vi "Bit Array to Number.vi"(0 "Bit 0":bool, 5 "Bit 1":bool, 7 "Bit 2":bool) -> (8 "flags":u16)   [LabVIEW 2014]
panel:
  # "Copyright 2014 Vidrio Technologies\nScanImage 5 software is licensed under the Apache License, Version 2.0 (the \"License\"); you may not use any files contained\nwithin the ScanImage 5 release except in compliance with the License. You may obtain a copy of the License at\n http://www.apache.org/licenses/LICENSE-2.0\nUnless required by applicable law or agreed to in writing, software distributed under the License is distributed on an\n\"AS IS\" BASIS, WITHOUT WARRANTIES OR CONDITIONS OF ANY KIND, either express or implied. See the License for the\n specific language governing permissions and limitations under the License."
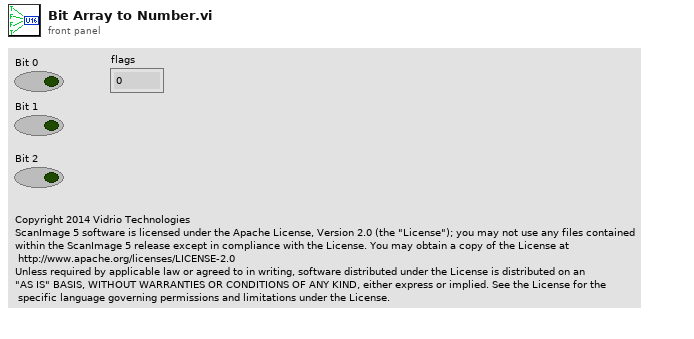
[diagram p1: front panel]
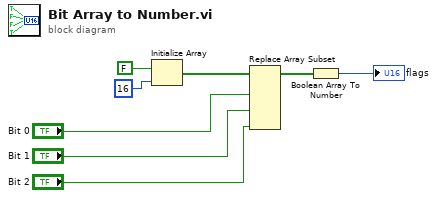
[diagram p0: block diagram]
diagram:
  n1 = Initialize Array(FALSE, 16 ("dimension size")) -> (w7:bool[])
  n2 = Replace Array Subset(array=w7, new element #1="Bit 0", new element #2="Bit 1", new element #3="Bit 2") -> (w5:bool[])  [unwired: 3 in]
  n3 = Boolean Array To Number(Boolean array=w5) -> (number=→"flags":u16)
